vi "AIMove.vi"(11 "input board":i32[][](array[numeric])) -> (3 "column":i32)   [LabVIEW 2025]
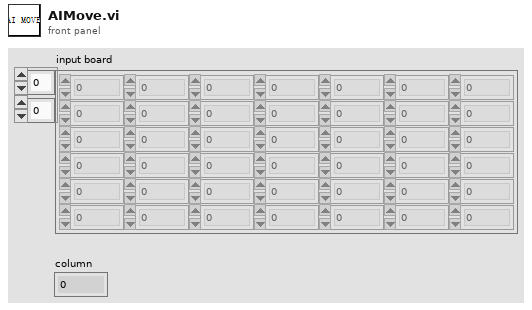
[diagram p1: front panel]
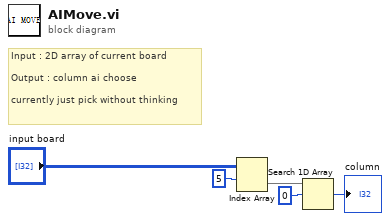
[diagram p0: block diagram]
diagram:
  # "Input : 2D array of current board\n\nOutput : column ai choose\n\ncurrently just pick without thinking"
  n1 = Index Array(array="input board", index (row)=5) -> (element=w3:i32[])  [unwired: 1 in]
  n2 = Search 1D Array(1D array=w3, element=0) -> (index of element=→"column":i32)  [unwired: 1 in]
